vi "BiasSpectroscopy.vi"() -> ()   [LabVIEW 2021]
doc: "Performs a Bias Spectroscopy with the option to apply several filters and display the numerical derivative of the output.\n\n- Nanonis Programming Interface -"
uses:
  Nanonis Prog Interface.lvlib
panel:
  in  "Filter order":i32=2 min=1 max=1000 step=1
  in  "Filter type":T1(ring)=enum."Gaussian"
  in  "Cutoff frq":dbl=0.125
  in  "Display":u16(ring)=1 items=["Y", "dY/dX", "dY/dX/(Y/X)"]
  in  "Z-Controller":T2 {"Switch off Delay (s)" min=0 max=100 format="%#_6p"; "TipLift (m)" format="%#_6p"}
  in  "Spectroscopy Parameter":cluster{"Start":dbl, "Stop":dbl, "# Points":i32}={"Start"=-2.0, "Stop"=2.0, "# Points"=256} {"# Points" min=2; "Stop" format="%1_3p"; "Start" format="%1_3p"}
  in  "Channels":i32[](listbox)=[0]
  out "SaveData":refnum<k4>
  in  "Save Data":bool
  out "Data":sgl[][](array[numeric])
  out "UpdateGraphs":refnum<k4>
  out "RunSpec":refnum<k4>
  out "Raw data":cluster{"X out":dbl[], sgl[]}(graph)
  in  "Channel":u16(ring) items=["Current (A)", "Input 2 (V)", "Bias (V)"]
  out "Processed data":cluster{"X out":dbl[], "Y out":dbl[]}(graph)
  in  "Run Spectroscopy":bool
  out "AllQuit":bool
  in  "stop":bool
  in  "Autosave Data":enum16{"no change", "on", "off"}(ring)
  # "Temporary Variables"
  # "Parameters"
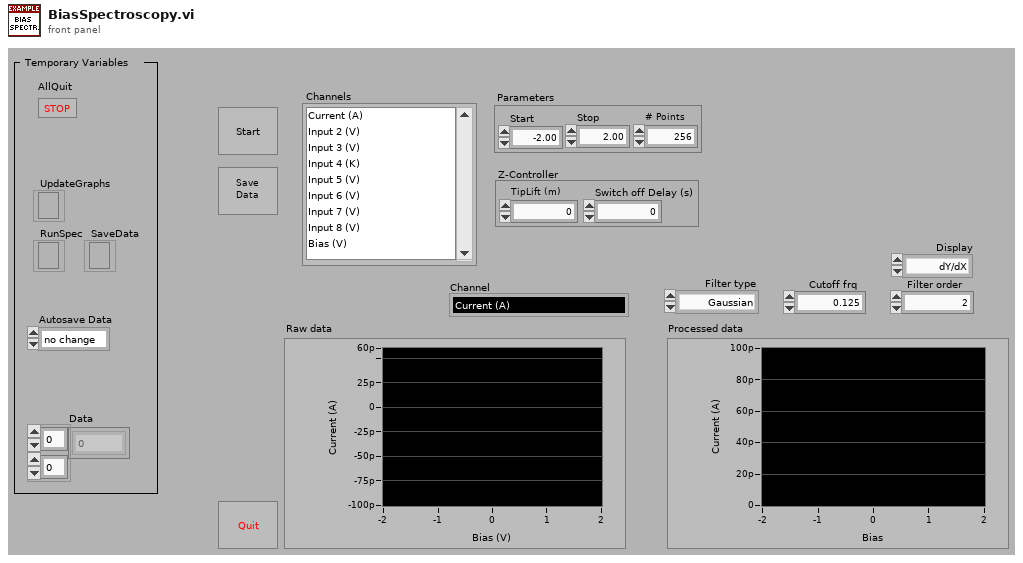
[diagram p1: front panel]
types:
  T1 = enum16{"none", "Gaussian", "Butterworth", "5th order FIR"}
  T2 = cluster{"TipLift (m)":dbl, "Switch off Delay (s)":sgl}
  T3 = cluster{"End settling time (s)":sgl, "Z control time (s)":sgl}
  T4 = cluster{"Z averaging time (s)":sgl, "Z offset (m)":sgl, "Initial settling time (s)":sgl}
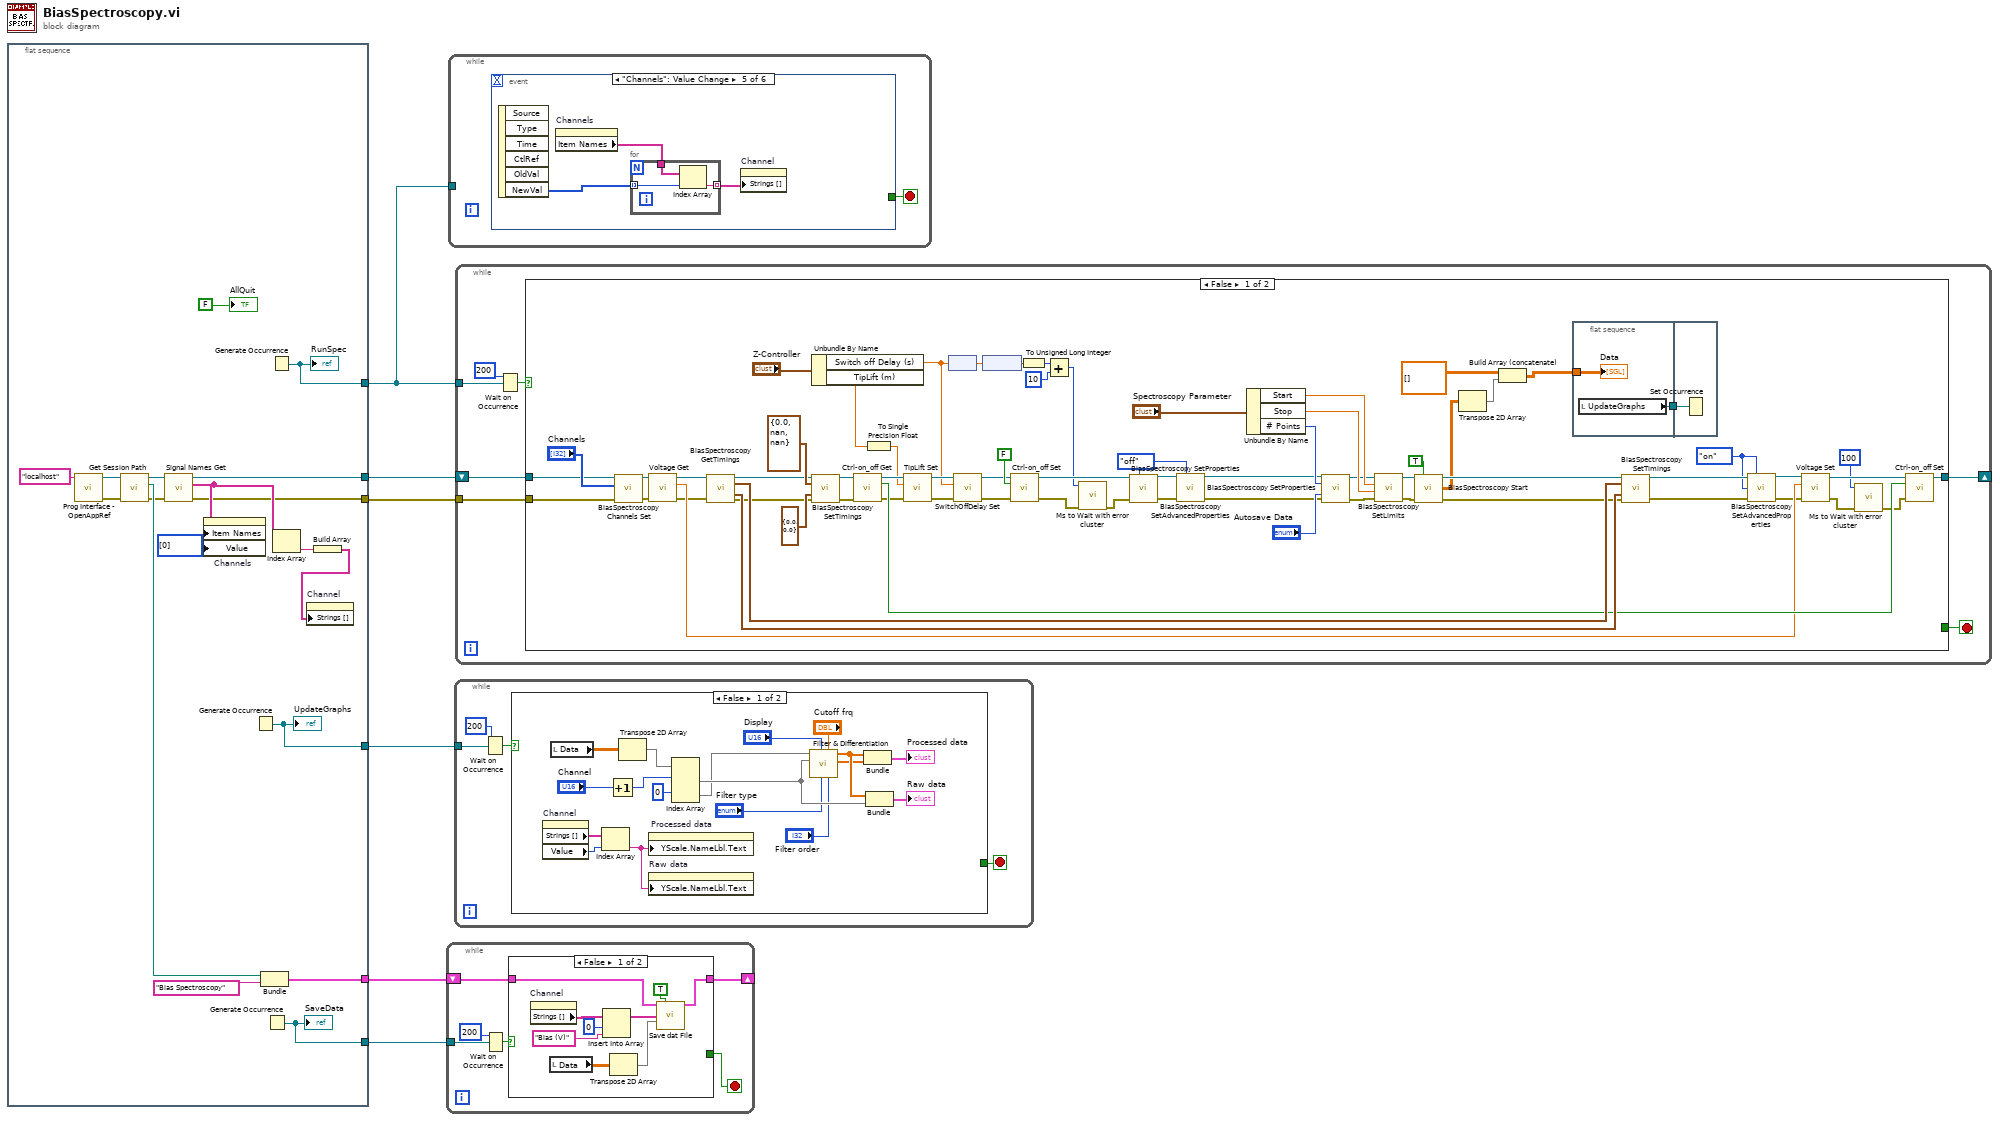
[diagram p0: block diagram]
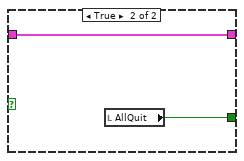
[diagram p2: hidden frame]
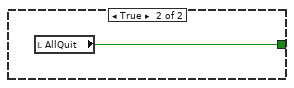
[diagram p3: hidden frame]
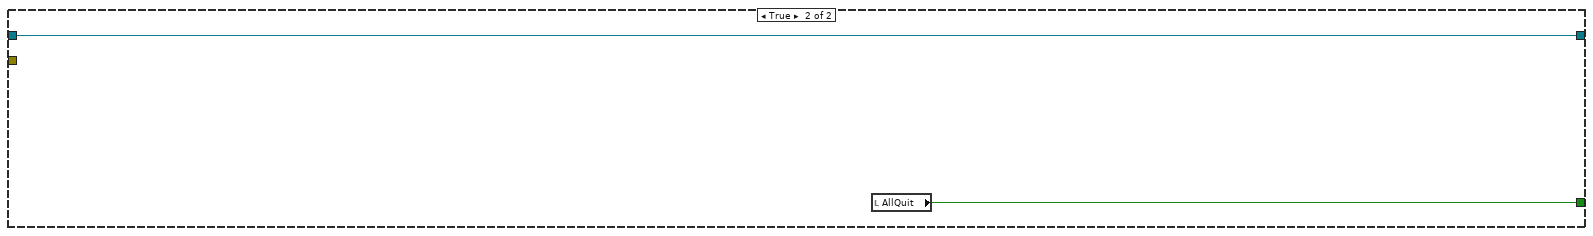
[diagram p4: hidden frame]
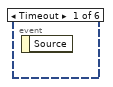
[diagram p5: hidden frame]
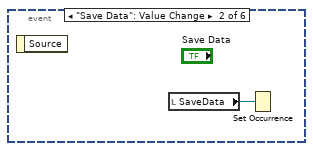
[diagram p6: hidden frame]
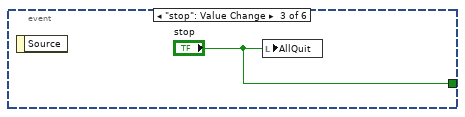
[diagram p7: hidden frame]
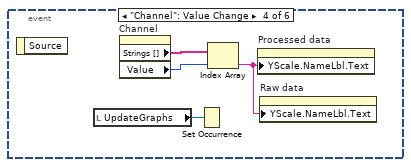
[diagram p8: hidden frame]
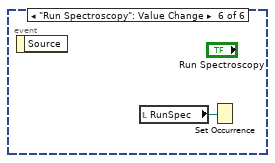
[diagram p9: hidden frame]
diagram:
  n1 = flat-sequence {
    tunnel: [w7] -> w6
    tunnel: [w20] -> w1
    tunnel: [w22] -> w5
    tunnel: [w21] -> w4
    tunnel: [w10] -> w3
    tunnel: [w15] -> w2
    frame #0 {
      n2 = call <userlib>:"Prog Interface - OpenAppRef.vi"("Machine name (local machine IP)"="localhost" ("Machine name (localhost)")) -> ("Error out"=w18:errorcluster, "Application reference"=w19:refnum<vi>)  [unwired: 5 in]
      n3 = call <userlib>:"Get Session Path.vi"("error in (no error)"=w18, "Application ref in"=w19) -> ("error out"=w8:errorcluster, "Session path"=w16:path, "Application ref out"=w11:refnum<vi>)  [unwired: 7 in]
      n4 = call <userlib>:"Signal Names Get.vi"("error in (no error)"=w8, "Application ref in"=w11) -> ("error out"=w7:errorcluster, "Signals Names"=w9:string[], "Application ref out"=w10:refnum<vi>)  [unwired: 5 in]
      n5 = property on="Channels" class="LstBox (strict)"("Item Names"=w9, "Value"=i32[] [0] ("Channels")) -> ()  [unwired: 2 in, 2 out]
      n6 = Generate Occurrence() -> (w22:refnum<k4>)
      "UpdateGraphs" <- w22
      n7 = Bundle("Session path"=w16, "Basename"="Bias Spectroscopy") -> (w15:cluster{"Session path":path, "Basename":string})  [unwired: 1 in]
      n8 = Generate Occurrence() -> (w21:refnum<k4>)
      "SaveData" <- w21
      n9 = Generate Occurrence() -> (w20:refnum<k4>)
      "RunSpec" <- w20
      n10 = Index Array(array=w9) -> (element=w13:string)  [unwired: 1 in]
      n11 = Build Array(w13) -> (w12:string[])
      n12 = property on="Channel" class="Ring (strict)"("Strings []"=w12) -> ()  [unwired: 2 in, 2 out]
      "AllQuit" <- FALSE ("AllQuit")
    }
  }
  n13 = while {
    tunnel: w4 -> [w28]
    shift-right: [w25] -> _
    shift-left: w2 -> [w26]
    stop <- w29 stop-if-true
    n14 = Wait on Occurrence(2:w28, 3:200 ("ms timeout (-1)")) -> (0:w30:bool)  [unwired: 1 in]
    n15 = case shown="False" w30 {
      tunnel: [_ w41] -> w29
      tunnel: w26 -> [w32 w40]
      tunnel: [w31 w40] -> w25
      frame False {
        n16 = property on="Channel" class="Ring (strict)"() -> ("Strings []"=w38:string[])  [unwired: 2 in, 2 out]
        n17 = local read "Data"() -> (w35:sgl[][])
        n18 = Insert Into Array(array=w38, index=0, new element="Bias (V)") -> (w36:string[])
        n19 = Transpose 2D Array(2D array=w35) -> (transposed array=w34:sgl[][])
        n20 = call <userlib>:"Save dat File.vi"("Filename control"=w32, "Show save dialog (T)"=TRUE, "Channels names"=w36, "Data"=w34) -> ("Filename control out"=w31:cluster{"Path":path, "Basename":string})  [unwired: 8 in, 3 out]
      }
      frame True {
        n21 = local read "AllQuit"() -> (w41:bool)
      }
    }
  }
  n22 = while {
    tunnel: w1 -> [_]
    stop <- w42 stop-if-true
    n23 = event shown="[4] \"Channels\": Value Change" {
      selector: _ -> [_ _ _ _ _ _]
      dyn-events: _ -> [_ _ _ _ _ _]
      timeout: _ -> [_ _ _ _ _ _]
      tunnel: [_ _ "stop" _ _ _] -> w42
      event Timeout {
        n24 = event-data() -> ()  [unwired: 1 in, 1 out]
      }
      event "Save Data": Value Change {
        n25 = event-data() -> ()  [unwired: 1 in, 1 out]
        n26 = local read "SaveData"() -> (w43:refnum<k4>)
        n27 = Set Occurrence(w43) -> ()
      }
      event "stop": Value Change {
        n28 = event-data() -> ()  [unwired: 1 in, 1 out]
        n29 = local write "AllQuit"("stop") -> ()
      }
      event "Channel": Value Change {
        n30 = event-data() -> ()  [unwired: 1 in, 1 out]
        n31 = local read "UpdateGraphs"() -> (w46:refnum<k4>)
        n32 = property on="Channel" class="Ring (strict)"() -> ("Strings []"=w48:string[], "Value"=w45:u16)  [unwired: 2 in, 2 out]
        n33 = Set Occurrence(w46) -> ()
        n34 = Index Array(array=w48, index=w45) -> (element=w47:string)
        n35 = property on="Processed data" class="XYGraph (strict)"("YScale.NameLbl.Text"=w47) -> ()  [unwired: 2 in, 2 out]
        n36 = property on="Raw data" class="XYGraph (strict)"("YScale.NameLbl.Text"=w47) -> ()  [unwired: 2 in, 2 out]
      }
      event "Channels": Value Change {
        n37 = event-data() -> ("NewVal"=w51:i32[])  [unwired: 1 in, 5 out]
        n38 = property on="Channels" class="LstBox (strict)"() -> ("Item Names"=w50:string[])  [unwired: 2 in, 2 out]
        n39 = for {
          tunnel: w51 -> [w53] mode=indexing
          tunnel: w50 -> [w54]
          tunnel: [w52] -> w49 mode=indexing
          n40 = Index Array(array=w54, index=w53) -> (element=w52:string)
        }
        n41 = property on="Channel" class="Ring (strict)"("Strings []"=w49) -> ()  [unwired: 2 in, 2 out]
      }
      event "Run Spectroscopy": Value Change {
        n42 = event-data() -> ()  [unwired: 1 in, 1 out]
        n43 = local read "RunSpec"() -> (w55:refnum<k4>)
        n44 = Set Occurrence(w55) -> ()
      }
    }
  }
  n45 = while {
    tunnel: w5 -> [w59]
    stop <- w56 stop-if-true
    n46 = Wait on Occurrence(2:w59, 3:200 ("ms timeout (-1)")) -> (0:w57:bool)  [unwired: 1 in]
    n47 = case shown="False" w57 {
      tunnel: [_ w78] -> w56
      frame False {
        n48 = property on="Channel" class="Ring (strict)"() -> ("Strings []"=w70:string[], "Value"=w69:u16)  [unwired: 2 in, 2 out]
        n49 = local read "Data"() -> (w76:sgl[][])
        n50 = Index Array(array=w70, index=w69) -> (element=w68:string)
        n51 = Increment(x="Channel") -> (x+1=w74:u16)
        n52 = Transpose 2D Array(2D array=w76) -> (transposed array=w75:sgl[][])
        n53 = property on="Processed data" class="XYGraph (strict)"("YScale.NameLbl.Text"=w68) -> ()  [unwired: 2 in, 2 out]
        n54 = property on="Raw data" class="XYGraph (strict)"("YScale.NameLbl.Text"=w68) -> ()  [unwired: 2 in, 2 out]
        n55 = Index Array(array=w75, index (row) #1=w74, index (row) #2=0 ("index (row)")) -> (element #1=w67:sgl[], element #2=w66:sgl[])  [unwired: 2 in]
        n56 = call <userlib>:"Filter & Differentiation.vi"("Filter order (2)"="Filter order", "Cutoff frq (0.125)"="Cutoff frq", "Filter type (none)"="Filter type", "Display (Y)"="Display", "Y in"=w67, "X in"=w66) -> ("Y out"=w64:dbl[], "X out"=w65:dbl[])  [unwired: 3 in, 1 out]
        n57 = Bundle("X out"=w65, "Y out"=w64) -> (→"Processed data":cluster{"X out":dbl[], "Y out":dbl[]})  [unwired: 1 in]
        n58 = Bundle("X out"=w65, w67) -> (→"Raw data":cluster{"X out":dbl[], sgl[]})  [unwired: 1 in]
      }
      frame True {
        n59 = local read "AllQuit"() -> (w78:bool)
      }
    }
  }
  n60 = while {
    tunnel: w6 -> [w85]
    tunnel: w1 -> [w84]
    shift-right: [w79] -> _
    shift-left: w3 -> [w80]
    stop <- w81 stop-if-true
    n61 = Wait on Occurrence(2:w84, 3:200 ("ms timeout (-1)")) -> (0:w82:bool)  [unwired: 1 in]
    n62 = case shown="False" w82 {
      tunnel: w85 -> [w112 _]
      tunnel: [_ w157] -> w81
      tunnel: w80 -> [w113 w156]
      tunnel: [w134 w156] -> w79
      frame False {
        w91 = enum16{"no change", "on", "off"}."on" ("Reset Bias (no change)")
        w86 = enum16{"no change", "on", "off"}."off" ("Reset Bias (no change)")
        n63 = call <userlib>:"BiasSpectroscopy Channels Set.vi"("Error in (no error)"=w112, "Channels"="Channels") -> ("Error out"=w100:errorcluster)  [unwired: 8 in, 1 out]
        n64 = call <userlib>:"Voltage Get.vi"("error in (no error)"=w100, "Application ref in"=w113) -> ("error out"=w138:errorcluster, "Bias (V)"=w143:sgl, "Application ref out"=w141:refnum<vi>)  [unwired: 7 in]
        n65 = call <userlib>:"BiasSpectroscopy GetTimings.vi"("Application ref in"=w141, "Error in (no error)"=w138) -> ("Application ref out"=w140:refnum<vi>, "Initialization"=w148:T4, "End of Sweep"=w147:T3, "Error out"=w137:errorcluster)  [unwired: 9 in, 1 out]
        n66 = Unbundle By Name("Z-Controller") -> ("Switch off Delay (s)"=w97:sgl, "TipLift (m)"=w96:dbl)
        n67 = call <userlib>:"BiasSpectroscopy SetTimings.vi"("Application ref in"=w140, "Initialization (NaN)"=T4 {"Z averaging time (s)"=0.0, "Z offset (m)"=nan, "Initial settling time (s)"=nan}, "End of Sweep (NaN)"=T3 {"End settling time (s)"=0.0, "Z control time (s)"=0.0}, "Error in (no error)"=w137) -> ("Application ref out"=w139:refnum<vi>, "Error out"=w136:errorcluster)  [unwired: 10 in]
        n68 = call <userlib>:"Ctrl-on_off Get.vi"("error in (no error)"=w136, "Application ref in"=w139) -> ("error out"=w127:errorcluster, "Z-Controller on/off status"=w144:bool, "Application ref out"=w128:refnum<vi>)  [unwired: 7 in]
        n69 = To Single Precision Float(number=w96) -> (single precision float=w123:sgl)
        n70 = call <userlib>:"TipLift Set.vi"("error in (no error)"=w127, "TipLift (m)"=w123, "Application ref in"=w128) -> ("error out"=w124:errorcluster, "Application ref out"=w126:refnum<vi>)  [unwired: 7 in]
        n71 = node(w97) -> (w122:sgl[unit])
        n72 = call <userlib>:"SwitchOffDelay Set.vi"("error in (no error)"=w124, "Switch off Delay (s)"=w97, "Application ref in"=w126) -> ("error out"=w117:errorcluster, "Application ref out"=w125:refnum<vi>)  [unwired: 7 in]
        n73 = node(w122) -> (w121:sgl)
        n74 = call <userlib>:"Ctrl-on_off Set.vi"("error in (no error)"=w117, "Z Controller ON/OFF"=FALSE, "Application ref in"=w125) -> ("error out"=w116:errorcluster, "Application ref out"=w133:refnum<vi>)  [unwired: 7 in]
        n75 = To Unsigned Long Integer(number=w121) -> (unsigned 32bit integer=w120:u32)
        n76 = Add(x=w120, y=u32 10) -> (x+y=w119:u32)
        n77 = call "Ms to Wait with error cluster.vi"("error in (no error)"=w116, "milliseconds to wait"=w119) -> ("error out"=w115:errorcluster)  [unwired: 4 in, 1 out]
        n78 = call <userlib>:"BiasSpectroscopy SetProperties.vi"("Application ref in"=w133, "Backward sweep (no change)"=w86, "Error in (no error)"=w115) -> ("Application ref out"=w90:refnum<vi>, "Error out"=w88:errorcluster)  [unwired: 11 in]
        n79 = call <userlib>:"BiasSpectroscopy SetAdvancedProperties.vi"("Application ref in"=w90, "Reset Bias (no change)"=w86, "Error in (no error)"=w88) -> ("Application ref out"=w89:refnum<vi>, "Error out"=w87:errorcluster)  [unwired: 11 in]
        n80 = Unbundle By Name("Spectroscopy Parameter") -> ("Start"=w105:dbl, "Stop"=w106:dbl, "# Points"=w99:i32)
        n81 = call <userlib>:"BiasSpectroscopy SetProperties.vi"("Application ref in"=w89, "Number of points (0=no change)"=w99, "Autosave (no change)"="Autosave Data", "Error in (no error)"=w87) -> ("Application ref out"=w104:refnum<vi>, "Error out"=w109:errorcluster)  [unwired: 10 in]
        n82 = call <userlib>:"BiasSpectroscopy SetLimits.vi"("Error in (no error)"=w109, "End value (V)"=w106, "Start value (V)"=w105, "Application ref in"=w104) -> ("Error out"=w110:errorcluster, "Application ref out"=w103:refnum<vi>)  [unwired: 4 in]
        n83 = call <userlib>:"BiasSpectroscopy Start.vi"("Application ref in"=w103, "Get data (F)"=TRUE, "Error in (no error)"=w110) -> ("Application ref out"=w142:refnum<vi>, "Data"=w108:sgl[][], "Error out"=w101:errorcluster)  [unwired: 8 in, 2 out]
        n84 = Transpose 2D Array(2D array=w108) -> (transposed array=w107:sgl[][])
        n85 = Build Array (concatenate)(sgl[][] [] ("Data"), w107) -> (w150:sgl[][])
        n86 = flat-sequence {
          tunnel: w150 -> [w154]
          tunnel: [w153] -> w149
          tunnel: w149 -> [w155]
          frame #0 {
            n87 = local read "UpdateGraphs"() -> (w153:refnum<k4>)
            "Data" <- w154
          }
          frame #1 {
            n88 = Set Occurrence(w155) -> ()
          }
        }
        n89 = call <userlib>:"BiasSpectroscopy SetTimings.vi"("Application ref in"=w142, "Initialization (NaN)"=w148, "End of Sweep (NaN)"=w147, "Error in (no error)"=w101) -> ("Application ref out"=w95:refnum<vi>, "Error out"=w94:errorcluster)  [unwired: 10 in]
        n90 = call <userlib>:"BiasSpectroscopy SetAdvancedProperties.vi"("Application ref in"=w95, "Reset Bias (no change)"=w91, "Record final Z (no change)"=w91, "Error in (no error)"=w94) -> ("Application ref out"=w93:refnum<vi>, "Error out"=w92:errorcluster)  [unwired: 10 in]
        n91 = call <userlib>:"Voltage Set.vi"("Error in (no error)"=w92, "Bias (V)"=w143, "Application ref in"=w93) -> ("Error out"=w131:errorcluster, "Application ref out"=w135:refnum<vi>)  [unwired: 7 in]
        n92 = call "Ms to Wait with error cluster.vi"("error in (no error)"=w131, "milliseconds to wait"=u32 100) -> ("error out"=w130:errorcluster)  [unwired: 4 in, 1 out]
        n93 = call <userlib>:"Ctrl-on_off Set.vi"("error in (no error)"=w130, "Z Controller ON/OFF"=w144, "Application ref in"=w135) -> ("Application ref out"=w134:refnum<vi>)  [unwired: 7 in, 1 out]
      }
      frame True {
        n94 = local read "AllQuit"() -> (w157:bool)
      }
    }
  }
